vi "single_measurements.vi"(8 "error in (no error)":errorcluster, 11 "UI in in":T1) -> (0 "error out":errorcluster, 2 "Measurement":dbl, 3 "UI out":T1)   [LabVIEW 2017]
uses:
  ui.ctl
  classes/dc_power_supply/DC_power_supply.lvclass
  ui_buttons.ctl
  types/boc_type.ctl
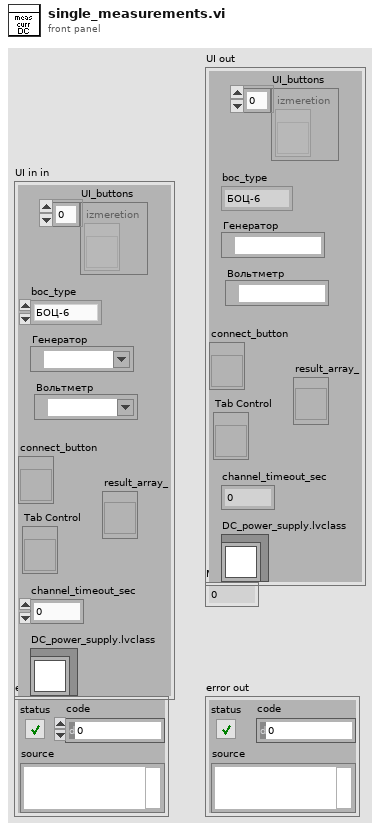
[diagram p1: front panel]
types:
  T1 = typedef "ui.ctl" = cluster{"UI_buttons":T2, "Tab Control":refnum<vi>, "connect_button":refnum<vi>, "generator":refnum<visa-resource-name>, "voltmetr":refnum<visa-resource-name>, "channel_timeout_sec":dbl, "boc_type":T3, "result_array_":refnum<vi>, "DC_power_supply.lvclass":refnum<class "DC_power_supply.lvclass">}
  T2 = typedef "ui_buttons.ctl" = refnum<vi>[]
  T3 = typedef "boc_type.ctl" = enum16{"БОЦ-6", "БОЦ-12"}
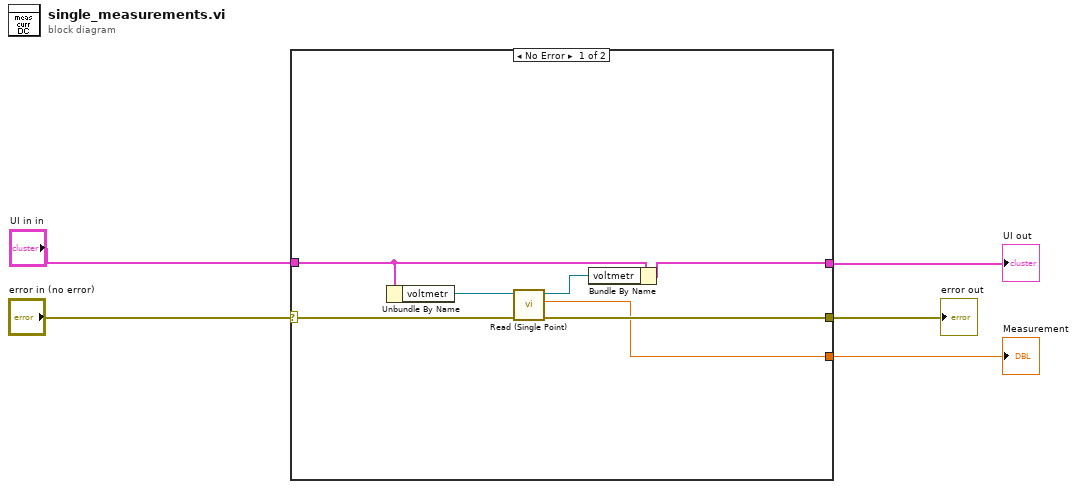
[diagram p0: block diagram]
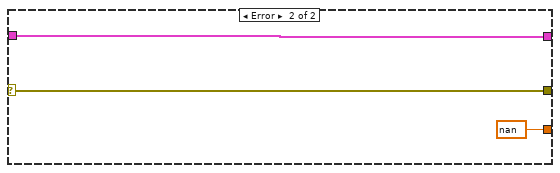
[diagram p2: hidden frame]
diagram:
  n1 = case shown="No Error" "error in (no error)" {
    selector: "error in (no error)" -> [w10 w15]
    tunnel: [w6 nan ("Measurement")] -> w2
    tunnel: [w7 w15] -> w3
    tunnel: "UI in in" -> [w11 w14]
    tunnel: [w12 w14] -> w1
    frame No Error {
      n2 = Unbundle By Name(w11) -> ("voltmetr"=w9:refnum<visa-resource-name>)
      n3 = call <instrlib>:"Read (Single Point).vi"("error in (no error)"=w10, "VISA resource name"=w9) -> ("error out"=w7:errorcluster, "Measurement"=w6:dbl, "VISA resource name out"=w8:refnum<visa-resource-name>)  [unwired: 7 in]
      n4 = Bundle By Name(cluster=w11, "voltmetr"=w8) -> (w12:T1)
    }
    frame Error {
    }
  }
  "Measurement" <- w2
  "error out" <- w3
  "UI out" <- w1
